vi "motor-XYZ-GlobalVar.vi"() -> ()   [LabVIEW 2014]
panel:
  in  "Z Position":dbl
  in  "Y Position":dbl
  in  "X Position":dbl
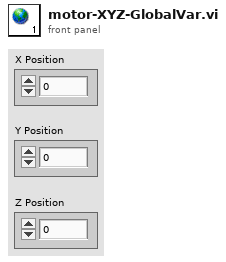
[diagram p1: front panel]
diagram:
